vi "Add NI-XNET Database.vi"(7 "Overwrite Existing?":bool=TRUE, 8 "error in (no error)":errorcluster, 9 "Database Alias":string, 10 "Base Node Path":string, 11 "SysDef Ref":T1) -> (0 "error out":errorcluster, 2 "New Node Path":string, 3 "SysDef Ref Out":T1)   [LabVIEW 2019, in "Simple SysDef API.lvlib"]
uses:
  <userlib>/SimpleSysDef/Simple SysDef API.lvlib
  <userlib>/SimpleSysDef/_SubVIs/System Definition Reference.ctl
  NationalInstruments.VeriStand.SystemDefinitionAPI
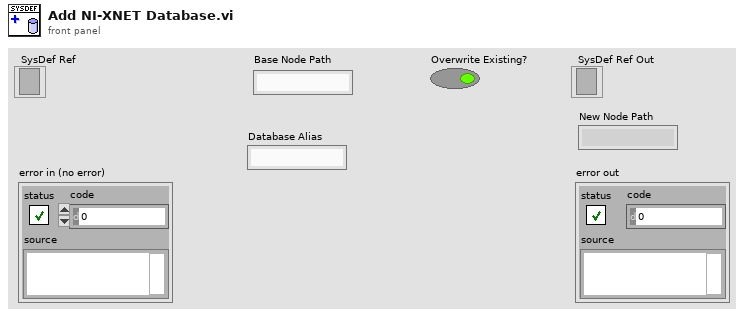
[diagram p1: front panel]
types:
  T1 = typedef "Simple SysDef API.lvlib/System Definition Reference.ctl" = refnum<k24>
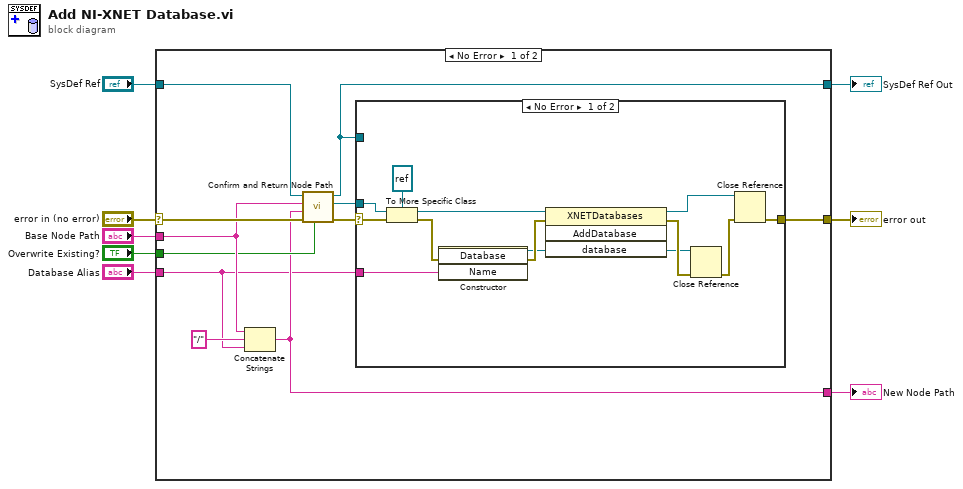
[diagram p0: block diagram]
diagram:
  n1 = case shown="No Error" "error in (no error)" {
    selector: "error in (no error)" -> [w19 w34]
    tunnel: [w16 w34] -> w7
    tunnel: "SysDef Ref" -> [w18 w33]
    tunnel: [w10 w33] -> w5
    tunnel: "Base Node Path" -> [w13 _]
    tunnel: "Overwrite Existing?" -> [w12 _]
    tunnel: [w11 _] -> w2
    tunnel: "Database Alias" -> [w9 _]
    frame No Error {
      n2 = Concatenate Strings(w13, "/" ("string"), w9) -> (w11:string)
      n3 = call <userlib>:"Confirm and Return Node Path.vi"("Overwrite Existing?"=w12, "error in (no error)"=w19, "New Node Path"=w11, "Base Node Path"=w13, "SysDef Ref"=w18) -> ("error out"=w14:errorcluster, "Node Ref"=w15:refnum<k24>, "SysDef Ref Out"=w10:T1)  [unwired: 4 in]
      n4 = case shown="No Error" w14 {
        selector: w14 -> [w30 w32]
        tunnel: [w29 w32] -> w16
        tunnel: w15 -> [w31 _]
        tunnel: w10 -> [_ _]
        tunnel: w9 -> [w20 _]
        frame No Error {
          n5 = To More Specific Class(target class=refnum<k24> refnum ("Node Ref"), reference=w31, error in=w30) -> (specific class reference=w27:refnum<k24>, error out=w26:errorcluster)
          n6 = constructor class="Database"(error in=w26, "Name"=w20) -> (reference out=w22:refnum<k24>, error out=w25:errorcluster)  [unwired: 2 in, 2 out]
          n7 = invoke class="XNETDatabases" method="AddDatabase"(reference=w27, error in=w25, "database"=w22) -> (reference out=w21:refnum<k24>, error out=w24:errorcluster)  [unwired: 1 in, 2 out]
          n8 = Close Reference(reference=w22, error in (no error)=w24) -> (error out=w23:errorcluster)
          n9 = Close Reference(reference=w21, error in (no error)=w23) -> (error out=w29:errorcluster)
        }
        frame Error {
        }
      }
    }
    frame Error {
    }
  }
  "SysDef Ref Out" <- w5
  "error out" <- w7
  "New Node Path" <- w2
